vi "Change_enum_typedef_strings.vi"(7 "Strings []":string[](array[string]), 10 "error in (no error)":errorcluster, 11 "protocol selection ref":refnum<vi>) -> (2 "error out":errorcluster)   [LabVIEW 2016]
uses:
  Typedef/Array_of_Comm_mode_and_address_types.ctl
  Typedef/Comm_mode_and_address_type.ctl
  Typedef/Comm_mode_type_combo.ctl
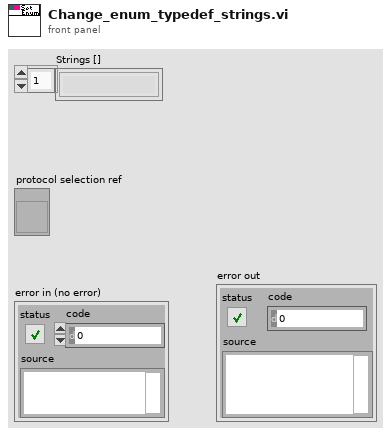
[diagram p1: front panel]
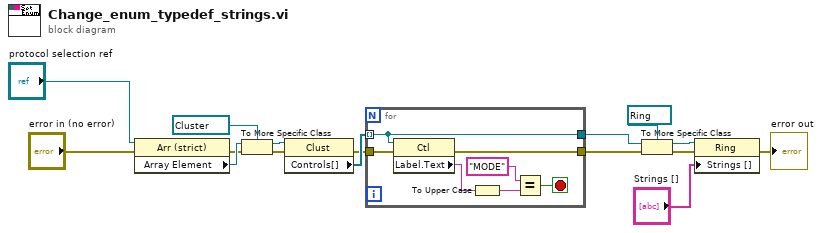
[diagram p0: block diagram]
diagram:
  n1 = property class="Arr (strict)"(reference="protocol selection ref", error in="error in (no error)") -> (error out=w3:errorcluster, "Array Element"=w12:refnum<vi>)  [unwired: 1 out]
  n2 = To More Specific Class(target class=refnum<vi> refnum ("Protocols"), reference=w12, error in=w3) -> (specific class reference=w10:refnum<vi>, error out=w2:errorcluster)
  n3 = property class="Clust"(reference=w10, error in=w2) -> (error out=w5:errorcluster, "Controls[]"=w9:refnum<vi>[])  [unwired: 1 out]
  n4 = for {
    tunnel: w9 -> [w19] mode=indexing
    tunnel: [w19] -> w8
    tunnel: w5 -> [w18]
    tunnel: [w17] -> w4
    stop <- w20 stop-if-true
    n5 = property class="Ctl"(reference=w19, error in=w18) -> (error out=w17:errorcluster, "Label.Text"=w23:string)  [unwired: 1 out]
    n6 = To Upper Case(1:w23) -> (0:w21:string)
    n7 = Equal?(x="MODE" ("all upper case string"), y=w21) -> (x = y?=w20:bool)
  }
  n8 = To More Specific Class(target class=refnum<vi> refnum ("Protocols"), reference=w8, error in=w4) -> (specific class reference=w15:refnum<vi>, error out=w14:errorcluster)
  n9 = property class="Ring"(reference=w15, error in=w14, "Strings []"="Strings []") -> (error out=→"error out":errorcluster)  [unwired: 1 out]
